vi "Add View.vi"(8 "error in (no error)":errorcluster, 10 "Debug Process":refnum<class "Debug View.lvclass">, 11 "Main In":refnum<class "Main.lvclass">) -> (0 "error out":errorcluster, 3 "Main Out":refnum<class "Main.lvclass">)   [LabVIEW 2020, in "Main.lvclass"]
uses:
  Main.lvclass
  Debug View/Debug View.lvclass
  Main.lvclass/Main.ctl
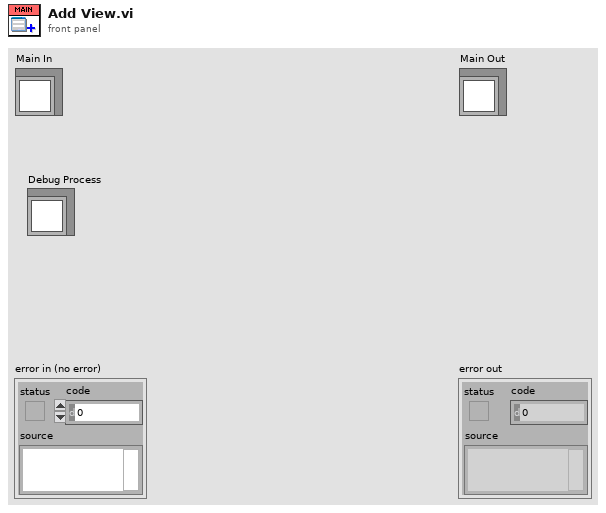
[diagram p1: front panel]
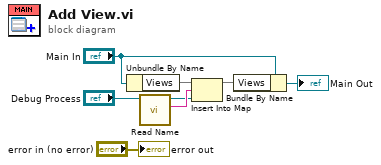
[diagram p0: block diagram]
diagram:
  n1 = Unbundle By Name("Main In") -> ("Views"=w4:map{string, refnum<class "Debug View.lvclass">})
  n2 = call "Read Name.vi"("Process In"="Debug Process") -> ("Name"=w2:string, "Process Out"=w1:refnum<class "Debug View.lvclass">)  [unwired: 8 in, 1 out]
  n3 = Insert Into Map(map in=w4, key=w2, value=w1) -> (map out=w3:map{string, refnum<class "Debug View.lvclass">})  [unwired: 2 out]
  n4 = Bundle By Name(cluster="Main In", "Views"=w3) -> (→"Main Out":refnum<class "Main.lvclass">)
  "error out" <- "error in (no error)"
